vi "Chronos TDMS File Viewer GUI.vi"(9 "ID":string, 10 "Default Time":T1, 11 "Default Channels":string[](array[string])) -> ()   [LabVIEW 2021]
uses:
  Viewer/cluster CC Channel from TDMS.ctl
  typedefs/Chronos cluster GUI Settings.ctl
  <vilib>/Utility/miscctls.llb/LVRangeTypeDef.ctl
  typedefs/Chronos cluster Current File.ctl
  typedefs/Chronos cluster Time Ranges.ctl
  Viewer/Chronos cluster Plot Settings.ctl
  GUI/Chronos cluster Map Limit Plots.ctl
  typedefs/Chronos cluster Plot Data and Limits.ctl
panel:
  in  "Channel Select":i32[](listbox)
  in  "reload":bool
  in  "Log Y":bool
  in  "Legend Visible":enum8{"False", "True", "Mixed"}(c332)
  in  "Y Autoscale":bool
  in  "X Autoscale":bool
  out "Loading...":string="LOADING..."
  out "XY Graph":cluster{dbl[], dbl[]}[](graph)
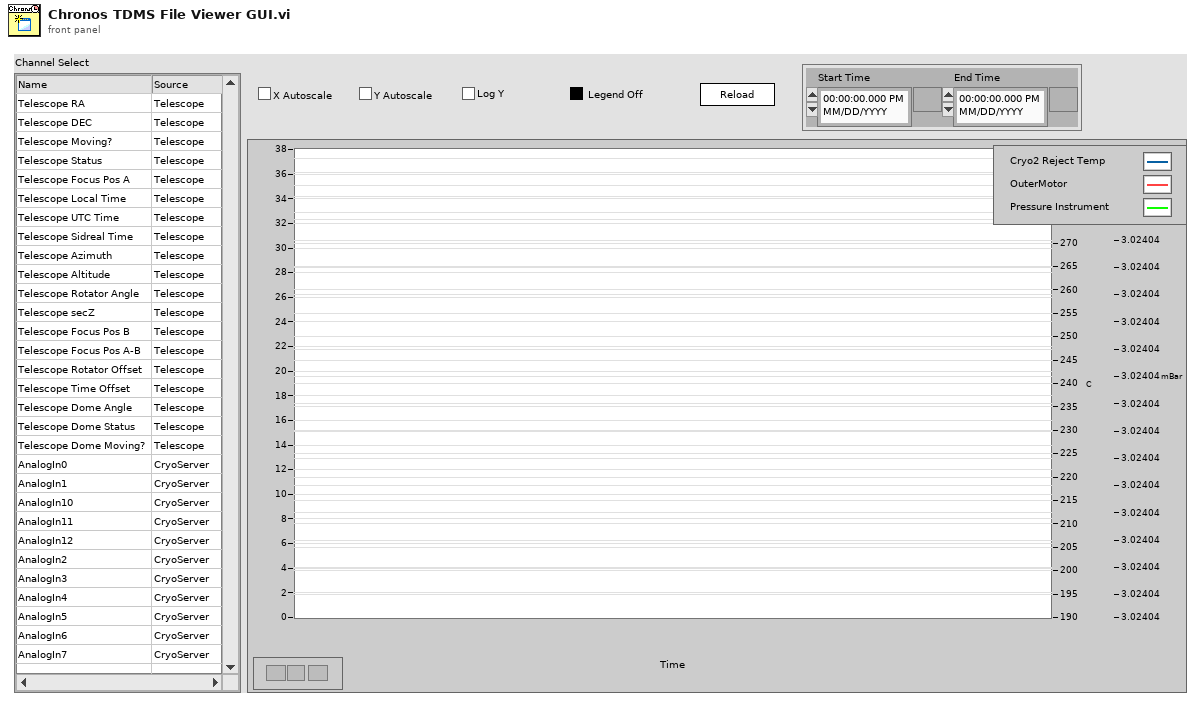
[diagram p1: front panel]
types:
  T1 = cluster{"Start Time":timestamp, "End Time":timestamp}
  T2 = typedef "cluster CC Channel from TDMS.ctl" = cluster{"Name":string, "Source":string, "Units":string}
  T3 = typedef "Chronos cluster GUI Settings.ctl" = cluster{"X Range":T4, "Select Ch":string[], "AutoScale":bool, "Show Limits":bool, "Path":path}
  T4 = typedef "LVRangeTypeDef.ctl" = cluster{"Minimum":dbl, "Maximum":dbl, "Increment":dbl, "Minor Increment":dbl, "Start":dbl}
  T5 = typedef "Chronos cluster Current File.ctl" = cluster{"path":path, "size":i64, "Plot Names":string[], "Offset":i32}
  T6 = typedef "Chronos cluster Time Ranges.ctl" = cluster{"Start Time":timestamp[], "End Time":timestamp[]}
  T7 = typedef "Chronos cluster Plot Settings.ctl" = cluster{"Plot Names":string[], "Colors":u32[], "Y Axis Indecies":i32[], "Units":string[], "Line Style":u8[]}
  T8 = typedef "Chronos cluster Map Limit Plots.ctl" = map{string, T9}
  T9 = typedef "Chronos cluster Plot Data and Limits.ctl" = cluster{"Data":cluster{dbl[], dbl[]}, "Data Units":string, "Limits":cluster{dbl[], dbl[]}[], "Limit Names":string[], "Channel":T2, "Group":string}
  T10 = cluster{"state":refnum<user-event>, "TDMS Files":path[], "Channel Names":string[], "Ch Data":T2[], "Settings":T3, "Current File":T5, "Time Ranges":T6, "Default Channels":string[], "Default Time":cluster{"Start Time":timestamp, "End Time":timestamp}, "Plot Attribs":T7, "Legend":enum8{"False", "True", "Mixed"}, "Plot":T8, "ID":string, "ch":T2}
  T11 = enum16{"open", "open or create", "create or replace", "create", "open (read-only)"}
  T12 = typedef "LVRectTypeDef.ctl" = cluster{"Left":i16, "Top":i16, "Right":i16, "Bottom":i16}
  T13 = typedef "Chronos cluster Viewer Window.ctl" = cluster{"Bounds":T12, "Channels":string[]}
  T14 = typedef "Chronos map Viewer Window List.ctl" = map{string, T13}
  T15 = enum32{"invalid app kind", "Development System", "Run Time System", "Student Edition", "Embedded LabVIEW", "Evaluation", "Custom"}
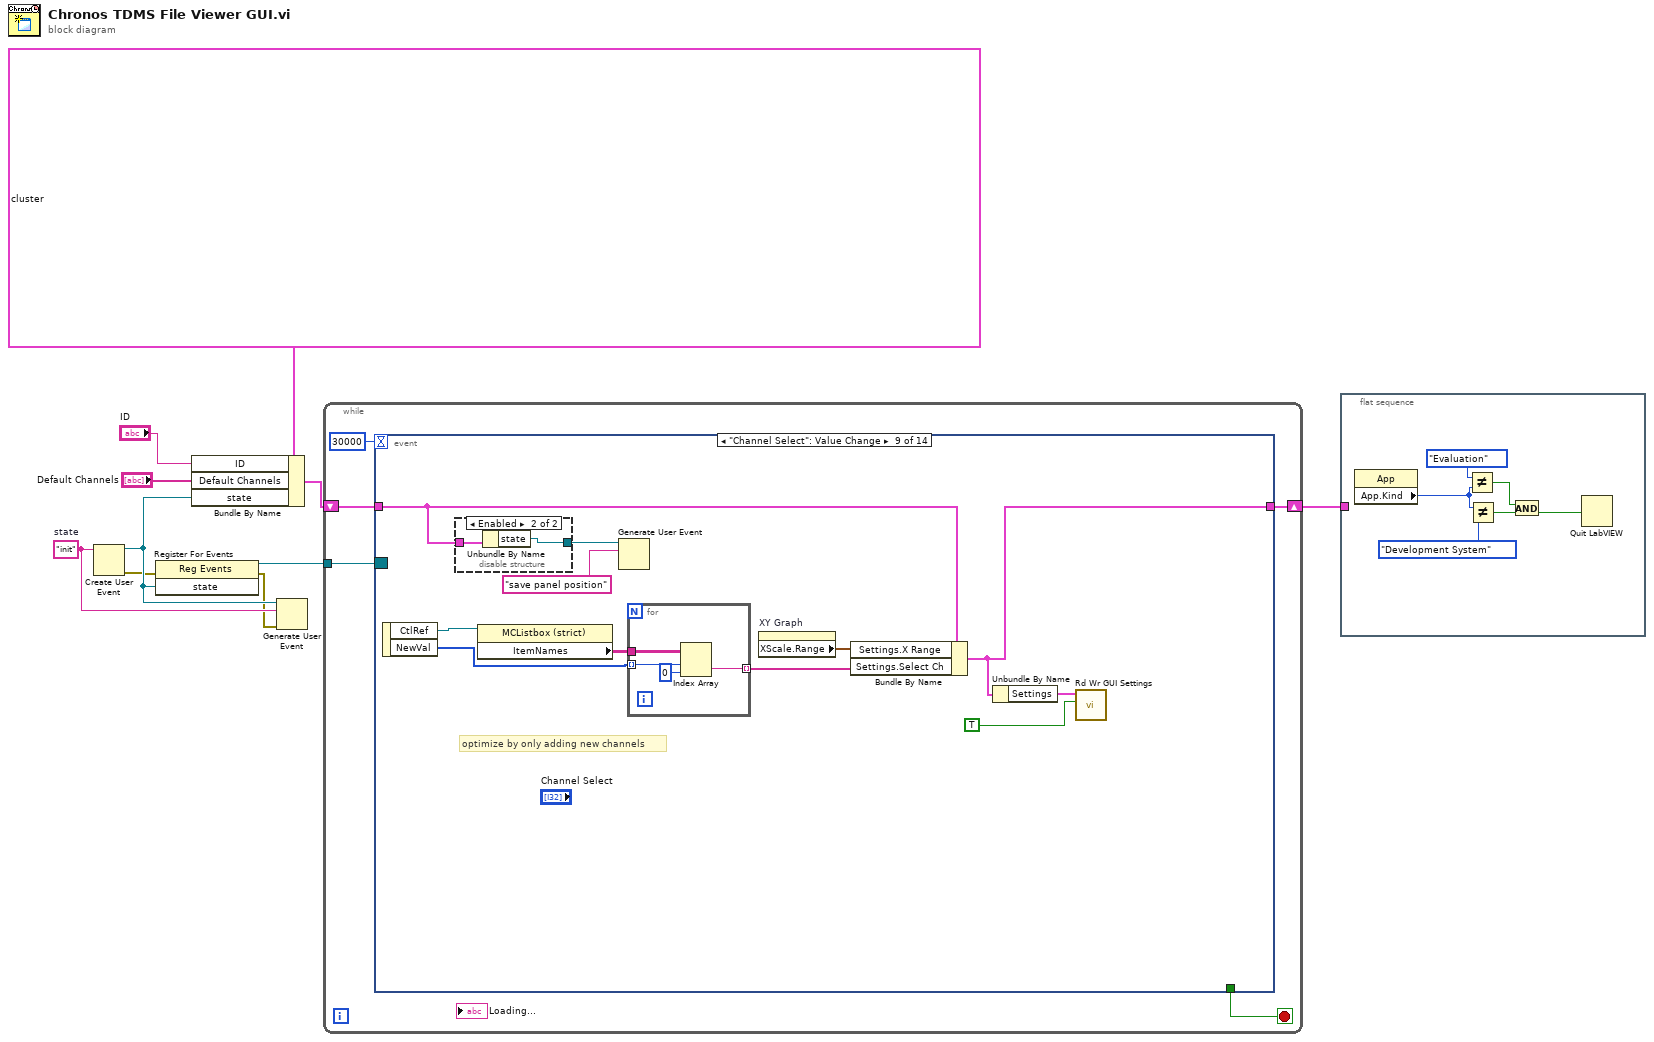
[diagram p0: block diagram]
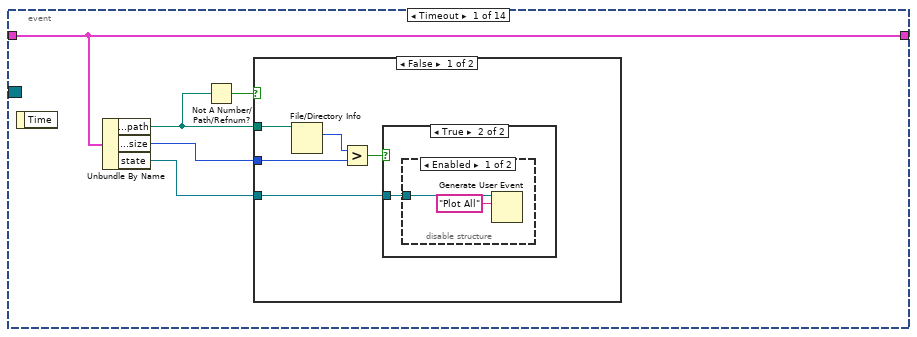
[diagram p2: hidden frame]
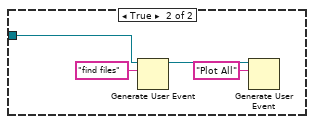
[diagram p5: hidden frame]
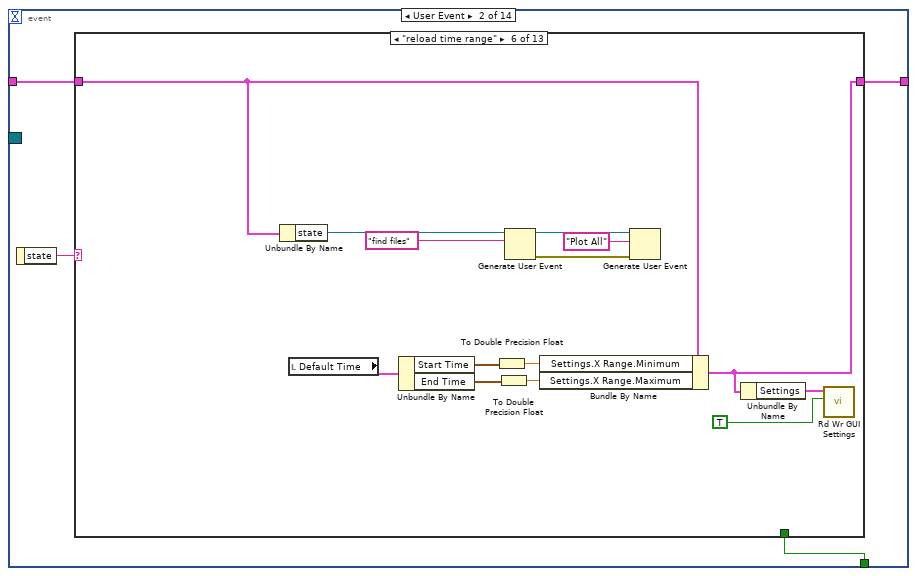
[diagram p6: hidden frame]
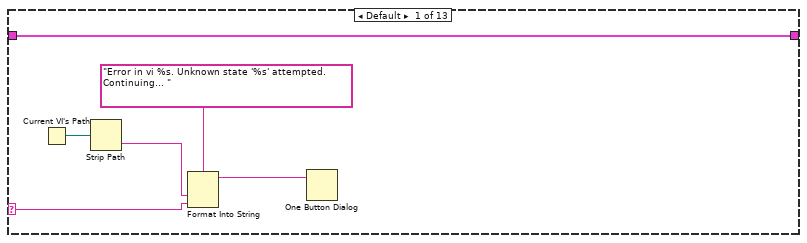
[diagram p7: hidden frame]
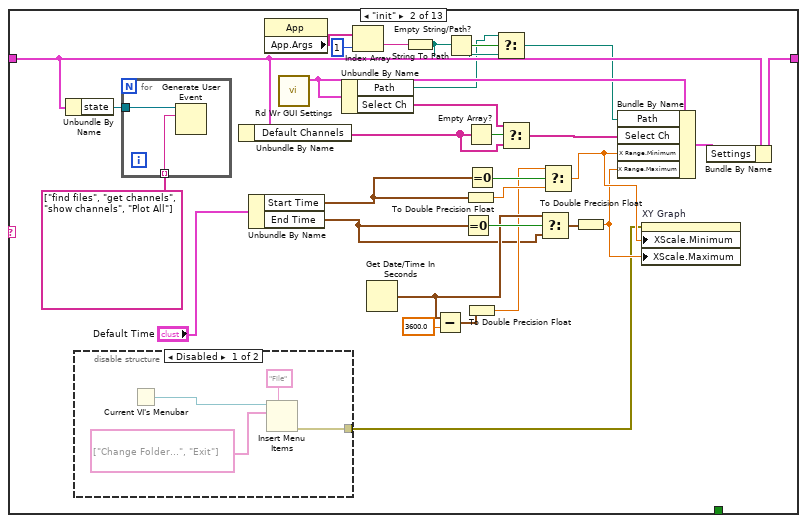
[diagram p8: hidden frame]
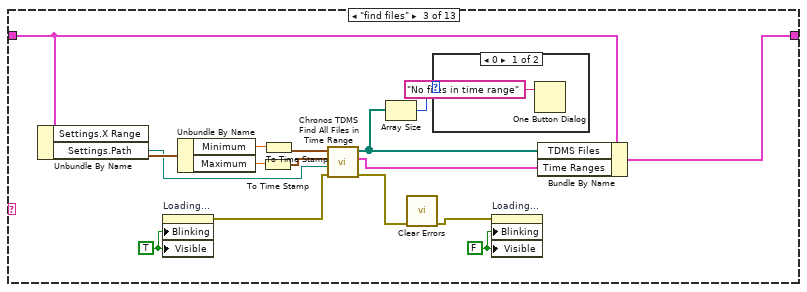
[diagram p10: hidden frame]
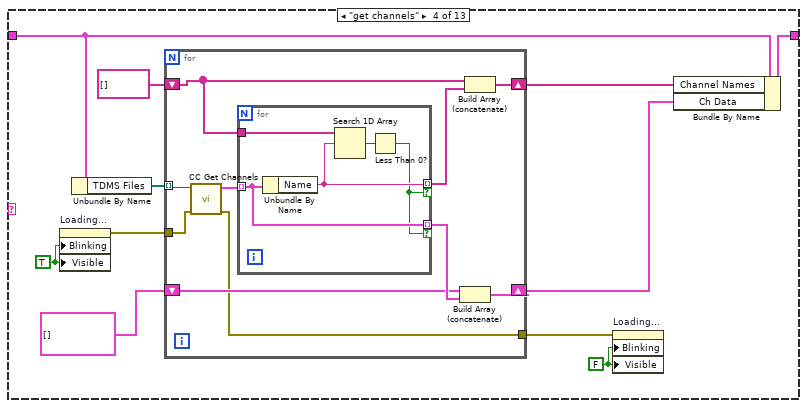
[diagram p12: hidden frame]
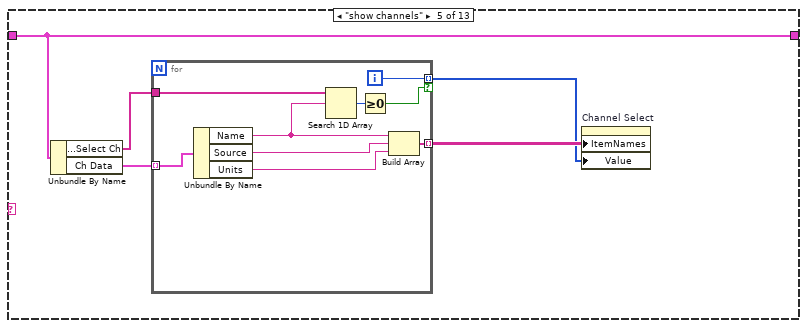
[diagram p13: hidden frame]
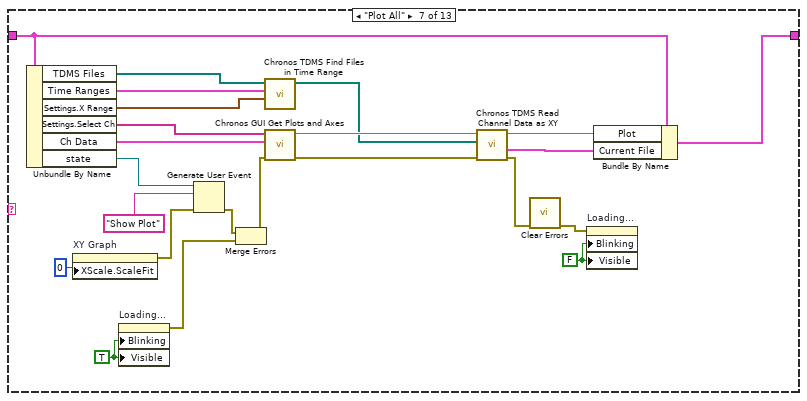
[diagram p14: hidden frame]
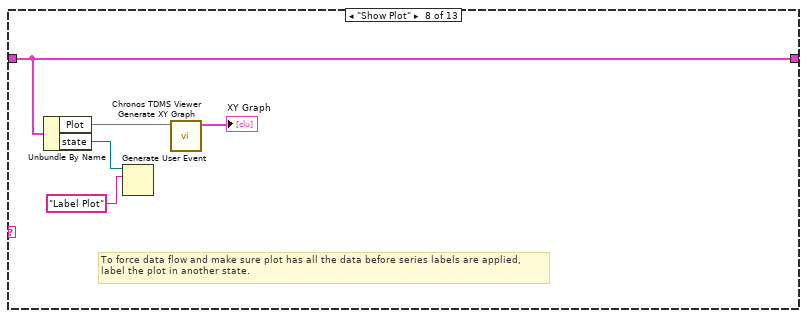
[diagram p15: hidden frame]
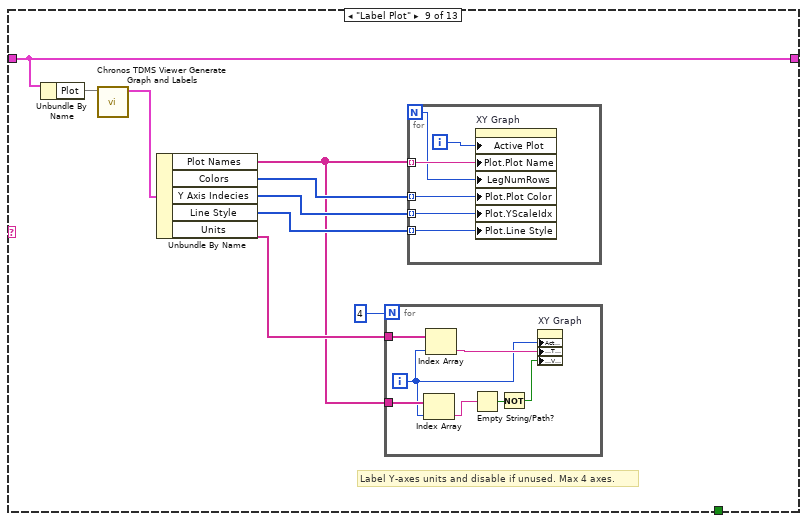
[diagram p16: hidden frame]
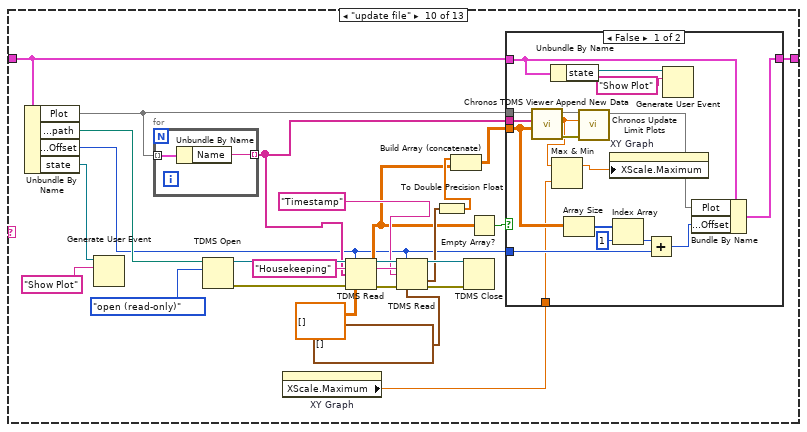
[diagram p17: hidden frame]
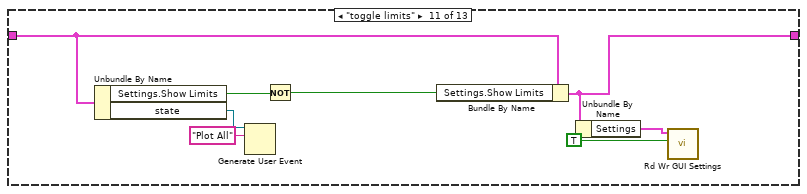
[diagram p19: hidden frame]
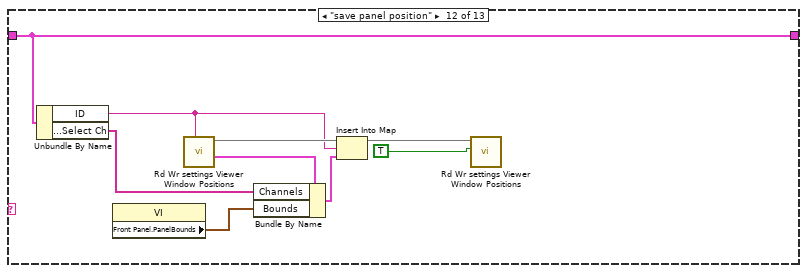
[diagram p20: hidden frame]
diagram:
  w6 = "init"  # state
  n1 = Create User Event(user event datatype=w6) -> (user event=w8:refnum<user-event>, error out=w4:errorcluster)  [unwired: 1 in]
  n2 = register-events(error in=w4, w8) -> (reference out=w7:refnum<event-registration>, error out=w5:errorcluster)  [unwired: 1 in]
  n3 = Bundle By Name(cluster=T10 {"state"=refnum, "TDMS Files"=[], "Channel Names"=[], "Ch Data"=[], "Settings"={"X Range"={"Minimum"=0.0, "Maximum"=0.0, "Increment"=0.0, "Minor Increment"=0.0, "Start"=0.0}, "Select Ch"=[], "AutoScale"=FALSE, "Show Limits"=FALSE, "Path"=path ""}, "Current File"={"path"=path "", "size"=0, "Plot Names"=[], "Offset"=0}, "Time Ranges"={"Start Time"=[], "End Time"=[]}, "Default Channels"=[], "Default Time"={"Start Time"=timestamp(0 s since 1904-01-01), "End Time"=timestamp(0 s since 1904-01-01)}, "Plot Attribs"={"Plot Names"=["Channel 02", "Channel 02 Red Low", "Channel 02 Red Hi", "Channel 02 Yellow Low", "Channel 02 Yellow Hi", "Channel 1", "Channel 1 Red Low", "Channel 1 Red Hi", "Channel 1 Yellow Low", "Channel 1 Yellow Hi"], "Colors"=[483491, 483491, 483491, 483491, 483491, 16728642, 16728642, 16728642, 16728642, 16728642], "Y Axis Indecies"=[0, 0, 0, 0, 0, 0, 0, 0, 0, 0], "Units"=["V"], "Line Style"=[]}, "Legend"=enum."False", "Plot"={}, "ID"="", "ch"={"Name"="", "Source"="", "Units"=""}}, "ID"="ID", "Default Channels"="Default Channels", "state"=w8) -> (w9:T10)
  n4 = Generate User Event(user event=w8, event data cluster=w6, error in=w5) -> ()  [unwired: 1 in, 2 out]
  n5 = while {
    tunnel: w7 -> [w15]
    shift-right: [w13] -> w1
    shift-left: w9 -> [w14]
    stop <- w12 stop-if-true
    n6 = event shown="[8] \"Channel Select\": Value Change" {
      selector: w15 -> [_ _ _ _ _ _ _ _ _ _ _ _ _ _]
      dyn-events: _ -> [_ _ _ _ _ _ _ _ _ _ _ _ _ _]
      timeout: 30000 -> [_ _ _ _ _ _ _ _ _ _ _ _ _ _]
      tunnel: w14 -> [w20 w35 w274 w313 w316 w318 w323 w327 w354 w374 w379 w385 w387 w393]
      tunnel: [w20 w34 w275 w313 w316 w318 w323 w328 w351 w374 w379 w385 w388 w393] -> w13
      tunnel: [_ w33 _ _ _ _ _ _ _ _ _ _ _ TRUE ("Close")] -> w12
      event Timeout {
        n7 = event-data() -> ()  [unwired: 1 in, 1 out]
        n8 = Unbundle By Name(w20) -> ("Current File.path"=w18:path, "Current File.size"=w17:i64, "state"=w16:refnum<user-event>)
        n9 = Not A Number/Path/Refnum?(number/path/refnum=w18) -> (NaN/Path/Refnum?=w19:bool)
        n10 = case shown="False" w19 {
          tunnel: w18 -> [w25 _]
          tunnel: w17 -> [w23 _]
          tunnel: w16 -> [w22 w31]
          frame False {
            n11 = File/Directory Info(path=w25) -> (size=w24:i64)  [unwired: 1 in, 6 out]
            n12 = Greater?(x=w24, y=w23) -> (0:w21:bool)
            n13 = case shown="True" w21 {
              tunnel: w22 -> [_ w26]
              frame False {
              }
              frame True {
                n14 = disable-structure shown="Enabled" {
                  disable-tunnel: w26 -> [w28 _]
                  frame Enabled {
                    n15 = Generate User Event(user event=w28, event data cluster="Plot All" ("event data")) -> ()  [unwired: 2 in, 2 out]
                  }
                  frame Disabled {
                  }
                }
              }
            }
          }
          frame True {
            n16 = Generate User Event(user event=w31, event data cluster="find files" ("event data")) -> (user event out=w30:refnum<user-event>)  [unwired: 2 in, 1 out]
            n17 = Generate User Event(user event=w30, event data cluster="Plot All" ("event data")) -> ()  [unwired: 2 in, 2 out]
          }
        }
      }
      event User Event {
        n18 = event-data() -> ("state"=w36:string)  [unwired: 1 in]
        n19 = case shown="\"reload time range\"" w36 {
          selector: w36 -> [w41 _ _ _ _ _ _ _ _ _ _ _ _]
          tunnel: w35 -> [w37 w69 w94 w104 w127 w143 w171 w178 w181 w218 w248 w263 w265]
          tunnel: [w37 w71 w95 w105 w127 w142 w172 w178 w181 w219 w249 w263 w265] -> w34
          tunnel: [_ _ _ _ _ _ _ _ _ _ _ _ TRUE] -> w33
          frame Default {
            n20 = Current VI's Path() -> (path=w40:path)
            n21 = Strip Path(path=w40) -> (name=w39:string)  [unwired: 1 out]
            n22 = Format Into String(format string="Error in vi %s. Unknown state '%s' attempted. Continuing... ", w39, w41) -> (resulting string=w38:string)  [unwired: 2 in, 1 out]
            n23 = One Button Dialog(message=w38) -> ()  [unwired: 1 in, 1 out]
          }
          frame "init" {
            n24 = Unbundle By Name(w69) -> ("state"=w73:refnum<user-event>)
            n25 = disable-structure shown="Disabled" {
              disable-tunnel: [w74 _] -> w43
              frame Disabled {
                n26 = Current VI's Menubar() -> (w77:refnum<k9>)
                n27 = Insert Menu Items(5:"File" ("menu tag"), 8:string[] ["Change Folder...", "Exit"] ("item names"), 9:w77) -> (0:w74:errorcluster)  [unwired: 3 in, 2 out]
              }
              frame Enabled {
              }
            }
            n28 = for {
              tunnel: w73 -> [w79]
              tunnel: string[] ["find files", "get channels", "show channels", "Plot All"] -> [w78] mode=indexing
              n29 = Generate User Event(user event=w79, event data cluster=w78) -> ()  [unwired: 2 in, 2 out]
            }
            n30 = Unbundle By Name(w69) -> ("Default Channels"=w64:string[])
            n31 = Unbundle By Name("Default Time") -> ("Start Time"=w45:timestamp, "End Time"=w44:timestamp)
            n32 = property class="App"() -> ("App.Args"=w53:string[])  [unwired: 2 in, 2 out]
            n33 = call "Rd Wr GUI Settings.vi"() -> ("Settings"=w68:T3)  [unwired: 10 in, 1 out]
            n34 = Unbundle By Name(w68) -> ("Path"=w49:path, "Select Ch"=w66:string[])
            n35 = Index Array(array=w53, index=1) -> (element=w51:string)
            n36 = Get Date/Time In Seconds() -> (seconds since 1Jan1904=w57:timestamp)
            n37 = String To Path(string=w51) -> (path=w50:path)
            n38 = Subtract(x=w57, y=3600.0) -> (x-y=w55:timestamp)
            n39 = Empty String/Path?(string/path=w50) -> (empty?=w52:bool)
            n40 = Equal To 0?(x=w44) -> (x = 0?=w62:bool)
            n41 = Empty Array?(array=w64) -> (empty?=w67:bool)
            n42 = To Double Precision Float(number=w45) -> (double precision float=w60:dbl)
            n43 = Equal To 0?(x=w45) -> (x = 0?=w63:bool)
            n44 = To Double Precision Float(number=w55) -> (double precision float=w54:dbl)
            n45 = Select(t=w49, s=w52, f=w50) -> (s? t:f=w48:path)
            n46 = Select(t=w66, s=w67, f=w64) -> (s? t:f=w65:string[])
            n47 = Select(t=w57, s=w62, f=w44) -> (s? t:f=w61:timestamp)
            n48 = Select(t=w54, s=w63, f=w60) -> (s? t:f=w59:dbl)
            n49 = To Double Precision Float(number=w61) -> (double precision float=w58:dbl)
            n50 = Bundle By Name(cluster=w68, "Path"=w48, "Select Ch"=w65, "X Range.Minimum"=w59, "X Range.Maximum"=w58) -> (w70:T3)
            n51 = property on="XY Graph" class="XYGraph (strict)"(error in=w43, "XScale.Minimum"=w59, "XScale.Maximum"=w58) -> ()  [unwired: 1 in, 2 out]
            n52 = Bundle By Name(cluster=w69, "Settings"=w70) -> (w71:T10)
          }
          frame "find files" {
            w85 = FALSE ("Visible")
            w87 = TRUE ("Visible")
            n53 = Unbundle By Name(w94) -> ("Settings.X Range"=w89:T4, "Settings.Path"=w82:path)
            n54 = property on="Loading..." class="Str"("Blinking"=w87, "Visible"=w87) -> (error out=w86:errorcluster)  [unwired: 2 in, 1 out]
            n55 = Unbundle By Name(w89) -> ("Minimum"=w93:dbl, "Maximum"=w92:dbl)
            n56 = To Time Stamp(1:w92) -> (0:w90:timestamp)
            n57 = To Time Stamp(1:w93) -> (0:w91:timestamp)
            n58 = call "Chronos TDMS Find All Files in Time Range.vi"("error in (no error)"=w86, "path"=w82, "End Time"=w90, "Start Time"=w91) -> ("error out"=w84:errorcluster, "Time Ranges"=w88:T6, "Files"=w81:path[])  [unwired: 5 in]
            n59 = Array Size(array=w81) -> (size(s)=w80:i32)
            n60 = call <vilib>:"Clear Errors.vi"("error in (no error)"=w84) -> ("error out"=w83:errorcluster)  [unwired: 5 in, 1 out]
            n61 = case shown="0" w80 {
              frame 0 {
                n62 = One Button Dialog(message="No files in time range") -> ()  [unwired: 1 in, 1 out]
              }
              frame 1, Default {
              }
            }
            n63 = property on="Loading..." class="Str"(error in=w83, "Blinking"=w85, "Visible"=w85) -> ()  [unwired: 1 in, 2 out]
            n64 = Bundle By Name(cluster=w94, "TDMS Files"=w81, "Time Ranges"=w88) -> (w95:T10)
          }
          frame "get channels" {
            w98 = FALSE ("Visible")
            w100 = TRUE ("Visible")
            n65 = property on="Loading..." class="Str"("Blinking"=w100, "Visible"=w100) -> (error out=w99:errorcluster)  [unwired: 2 in, 1 out]
            n66 = Unbundle By Name(w104) -> ("TDMS Files"=w107:path[])
            n67 = for {
              tunnel: w107 -> [w111] mode=indexing
              shift-right: [w117] -> w103
              shift-left: string[] [] -> [w116]
              shift-right: [w114] -> w101
              shift-left: T2[] [] -> [w112]
              tunnel: w99 -> [w109]
              tunnel: [w108] -> w97
              n68 = call "CC Get Channels.vi"("error in (no error)"=w109, "file path"=w111) -> ("error out"=w108:errorcluster, "Channel List"=w110:T2[])  [unwired: 8 in]
              n69 = for {
                tunnel: w110 -> [w119] mode=indexing
                tunnel: w116 -> [w122]
                tunnel: [w120] -> w115 mode=indexing if=w118
                tunnel: [w119] -> w113 mode=indexing if=w118
                n70 = Unbundle By Name(w119) -> ("Name"=w120:string)
                n71 = Search 1D Array(1D array=w122, element=w120) -> (index of element=w121:i32)  [unwired: 1 in]
                n72 = Less Than 0?(x=w121) -> (x < 0?=w118:bool)
              }
              n73 = Build Array (concatenate)(w112, w113) -> (w114:T2[])
              n74 = Build Array (concatenate)(w116, w115) -> (w117:string[])
            }
            n75 = property on="Loading..." class="Str"(error in=w97, "Blinking"=w98, "Visible"=w98) -> ()  [unwired: 1 in, 2 out]
            n76 = Bundle By Name(cluster=w104, "Channel Names"=w103, "Ch Data"=w101) -> (w105:T10)
          }
          frame "show channels" {
            n77 = Unbundle By Name(w127) -> ("Settings.Select Ch"=w124:string[], "Ch Data"=w126:T2[])
            n78 = for {
              tunnel: w126 -> [w136] mode=indexing
              tunnel: [w135] -> w125 mode=indexing
              tunnel: w124 -> [w134]
              tunnel: [w131] -> w123 mode=indexing if=w130
              i -> [w131]
              n79 = Unbundle By Name(w136) -> ("Name"=w133:string, "Source"=w129:string, "Units"=w128:string)
              n80 = Search 1D Array(1D array=w134, element=w133) -> (index of element=w132:i32)  [unwired: 1 in]
              n81 = Greater Or Equal To 0?(x=w132) -> (x >= 0?=w130:bool)
              n82 = Build Array(w133, w129, w128) -> (w135:string[])
            }
            n83 = property on="Channel Select" class="MCListbox (strict)"("ItemNames"=w125, "Value"=w123) -> ()  [unwired: 2 in, 2 out]
          }
          frame "reload time range" {
            n84 = Unbundle By Name(w143) -> ("state"=w148:refnum<user-event>)
            n85 = local read "Default Time"() -> (w141:T1)
            n86 = Unbundle By Name(w141) -> ("Start Time"=w139:timestamp, "End Time"=w138:timestamp)
            n87 = To Double Precision Float(number=w139) -> (double precision float=w140:dbl)
            n88 = To Double Precision Float(number=w138) -> (double precision float=w137:dbl)
            n89 = Generate User Event(user event=w148, event data cluster="find files" ("event data")) -> (user event out=w146:refnum<user-event>, error out=w145:errorcluster)  [unwired: 2 in]
            n90 = Bundle By Name(cluster=w143, "Settings.X Range.Minimum"=w140, "Settings.X Range.Maximum"=w137) -> (w142:T10)
            n91 = Generate User Event(user event=w146, event data cluster="Plot All" ("event data"), error in=w145) -> ()  [unwired: 1 in, 2 out]
            n92 = Unbundle By Name(w142) -> ("Settings"=w150:T3)
            n93 = call "Rd Wr GUI Settings.vi"("Write? (F:Read)"=TRUE, "Settings"=w150) -> ()  [unwired: 8 in, 2 out]
          }
          frame "Plot All" {
            w153 = FALSE ("Visible")
            w157 = TRUE ("Visible")
            n94 = Unbundle By Name(w171) -> ("TDMS Files"=w173:path[], "Time Ranges"=w170:T6, "Settings.X Range"=w167:T4, "Settings.Select Ch"=w169:string[], "Ch Data"=w168:T2[], "state"=w166:refnum<user-event>)
            n95 = property on="XY Graph" class="XYGraph (strict)"("XScale.ScaleFit"=u8 0 ("X Scale.Scale Fit")) -> (error out=w159:errorcluster)  [unwired: 2 in, 1 out]
            n96 = property on="Loading..." class="Str"("Blinking"=w157, "Visible"=w157) -> (error out=w154:errorcluster)  [unwired: 2 in, 1 out]
            n97 = Generate User Event(user event=w166, event data cluster="Show Plot" ("event data"), error in=w159) -> (error out=w156:errorcluster)  [unwired: 1 in, 1 out]
            n98 = Merge Errors(w156, w154) -> (w155:errorcluster)
            n99 = call "Chronos TDMS Find Files in Time Range.vi"("Scale"=w167, "Time Ranges"=w170, "TDMS Files"=w173) -> ("Files out"=w162:path[])  [unwired: 7 in, 1 out]
            n100 = call "Chronos GUI Get Plots and Axes.vi"("error in (no error)"=w155, "Ch Data"=w168, "Select Ch"=w169) -> ("error out"=w163:errorcluster, "Plot Map"=w164:T8)  [unwired: 7 in]
            n101 = call "Chronos TDMS Read Channel Data as XY.vi"("error in (no error)"=w163, "Files"=w162, "Limit Plot Map"=w164) -> ("error out"=w152:errorcluster, "Current File"=w160:T5, "Plot Map out"=w161:T8)  [unwired: 6 in]
            n102 = call <vilib>:"Clear Errors.vi"("error in (no error)"=w152) -> ("error out"=w151:errorcluster)  [unwired: 5 in, 1 out]
            n103 = property on="Loading..." class="Str"(error in=w151, "Blinking"=w153, "Visible"=w153) -> ()  [unwired: 1 in, 2 out]
            n104 = Bundle By Name(cluster=w171, "Plot"=w161, "Current File"=w160) -> (w172:T10)
          }
          frame "Show Plot" {
            # "To force data flow and make sure plot has all the data before series labels are applied,\nlabel the plot in another state."
            n105 = Unbundle By Name(w178) -> ("Plot"=w175:T8, "state"=w177:refnum<user-event>)
            n106 = Generate User Event(user event=w177, event data cluster="Label Plot" ("event data")) -> ()  [unwired: 2 in, 2 out]
            n107 = call "Chronos TDMS Viewer Generate XY Graph.vi"("Limit Plot Map"=w175) -> ("XY Graph"=→"XY Graph":cluster{dbl[], dbl[]}[])  [unwired: 9 in, 1 out]
          }
          frame "Label Plot" {
            # "Label Y-axes units and disable if unused. Max 4 axes."
            n108 = Unbundle By Name(w181) -> ("Plot"=w182:T8)
            n109 = call "Chronos TDMS Viewer Generate Graph and Labels.vi"("Limit Plot Map"=w182) -> ("Plot Settings"=w180:T7)  [unwired: 9 in, 1 out]
            n110 = Unbundle By Name(w180) -> ("Plot Names"=w179:string[], "Colors"=w187:u32[], "Y Axis Indecies"=w186:i32[], "Line Style"=w184:u8[], "Units"=w185:string[])
            n111 = for {
              N: 4 -> [_]
              tunnel: w185 -> [w193]
              tunnel: w179 -> [w190]
              i -> [w189]
              n112 = Index Array(array=w190, index=w189) -> (element=w188:string)
              n113 = Index Array(array=w193, index=w189) -> (element=w194:string)
              n114 = Empty String/Path?(string/path=w188) -> (empty?=w192:bool)
              n115 = Not(x=w192) -> (.not. x?=w191:bool)
              n116 = property on="XY Graph" class="XYGraph (strict)"("ActYScl"=w189, "YScale.NameLbl.Text"=w194, "YScale.Visible"=w191) -> ()  [unwired: 2 in, 2 out]
            }
            n117 = for {
              N -> [w198]
              tunnel: w179 -> [w199] mode=indexing
              tunnel: w186 -> [w197] mode=indexing
              tunnel: w187 -> [w196] mode=indexing
              tunnel: w184 -> [w195] mode=indexing
              i -> [w200]
              n118 = property on="XY Graph" class="XYGraph (strict)"("Active Plot"=w200, "Plot.Plot Name"=w199, "LegNumRows"=w198, "Plot.Plot Color"=w196, "Plot.YScaleIdx"=w197, "Plot.Line Style"=w195) -> ()  [unwired: 2 in, 2 out]
            }
          }
          frame "update file" {
            n119 = Unbundle By Name(w218) -> ("Plot"=w220:T8, "Current File.path"=w225:path, "Current File.Offset"=w201:i32, "state"=w217:refnum<user-event>)
            n120 = Generate User Event(user event=w217, event data cluster="Show Plot" ("event data")) -> ()  [unwired: 2 in, 2 out]
            n121 = for {
              tunnel: w220 -> [w247] mode=indexing
              tunnel: [w246] -> w213 mode=indexing
              n122 = Unbundle By Name(w247) -> ("Name"=w246:string)
            }
            n123 = TDMS Open(10:T11."open (read-only)" ("operation (0:open)"), 11:w225) -> (0:w222:errorcluster, 3:w223:refnum<k34>)  [unwired: 5 in]
            n124 = property on="XY Graph" class="XYGraph (strict)"() -> ("XScale.Maximum"=w214:dbl)  [unwired: 2 in, 2 out]
            n125 = TDMS Read(0:w223, 1:w201, 5:"Housekeeping" ("group name in"), 7:w213, 11:w222, 12:dbl[][] []) -> (4:w212:refnum<k34>, 6:w211:string, 10:w203:dbl[][], 15:w210:errorcluster)  [unwired: 2 in, 2 out]
            n126 = TDMS Read(0:w212, 1:w201, 5:w211, 7:"Timestamp", 11:w210, 12:timestamp[] []) -> (4:w206:refnum<k34>, 10:w205:timestamp[], 15:w207:errorcluster)  [unwired: 2 in, 3 out]
            n127 = To Double Precision Float(number=w205) -> (double precision float=w204:dbl[])
            n128 = Build Array (concatenate)(w204, w203) -> (w202:dbl[][])
            n129 = TDMS Close(8:w207, 11:w206) -> ()  [unwired: 2 out]
            n130 = Empty Array?(array=w203) -> (empty?=w215:bool)
            n131 = case shown="False" w215 {
              tunnel: w220 -> [w244 _]
              tunnel: [w241 w245] -> w219
              tunnel: w218 -> [w234 w245]
              tunnel: w201 -> [w239 _]
              tunnel: w202 -> [w236 _]
              tunnel: w213 -> [w231 _]
              tunnel: w214 -> [w228 _]
              frame False {
                n132 = call "Chronos TDMS Viewer Append New Data.vi"("data"=w236, "Ch Names"=w231, "Plot"=w244) -> ("error out"=w243:errorcluster, "end time"=w230:dbl, "Plot out"=w242:T8)  [unwired: 6 in]
                n133 = Unbundle By Name(w234) -> ("state"=w233:refnum<user-event>)
                n134 = Max & Min(x=w230, y=w228) -> (max(x,y)=w229:dbl)  [unwired: 1 out]
                n135 = Array Size(array=w236) -> (size(s)=w240:i32[])
                n136 = call "Chronos Update Limit Plots.vi"("error in (no error)"=w243, "End Time"=w230, "Limits"=w242) -> ("Limits out"=w235:T8)  [unwired: 7 in, 1 out]
                n137 = property on="XY Graph" class="XYGraph (strict)"("XScale.Maximum"=w229) -> ()  [unwired: 2 in, 2 out]
                n138 = Index Array(array=w240, index=1) -> (element=w227:i32)
                n139 = Add(x=w227, y=w239) -> (x+y=w238:i32)
                n140 = Generate User Event(user event=w233, event data cluster="Show Plot" ("event data")) -> ()  [unwired: 2 in, 2 out]
                n141 = Bundle By Name(cluster=w234, "Plot"=w235, "Current File.Offset"=w238) -> (w241:T10)
              }
              frame True {
              }
            }
          }
          frame "toggle limits" {
            n142 = Unbundle By Name(w248) -> ("Settings.Show Limits"=w255:bool, "state"=w253:refnum<user-event>)
            n143 = Generate User Event(user event=w253, event data cluster="Plot All" ("event data")) -> ()  [unwired: 2 in, 2 out]
            n144 = Not(x=w255) -> (.not. x?=w254:bool)
            n145 = Bundle By Name(cluster=w248, "Settings.Show Limits"=w254) -> (w249:T10)
            n146 = Unbundle By Name(w249) -> ("Settings"=w251:T3)
            n147 = call "Rd Wr GUI Settings.vi"("Write? (F:Read)"=TRUE, "Settings"=w251) -> ()  [unwired: 8 in, 2 out]
          }
          frame "save panel position" {
            n148 = Unbundle By Name(w263) -> ("ID"=w262:string, "Settings.Select Ch"=w259:string[])
            n149 = property class="VI"() -> ("Front Panel.PanelBounds"=w260:T12)  [unwired: 2 in, 2 out]
            n150 = call "Rd Wr settings Viewer Window Positions.vi"("Window name"=w262) -> ("value"=w261:T13, "Window Map"=w264:T14)  [unwired: 7 in, 2 out]
            n151 = Bundle By Name(cluster=w261, "Channels"=w259, "Bounds"=w260) -> (w256:T13)
            n152 = Insert Into Map(map in=w264, key=w262, value=w256) -> (map out=w258:T14)  [unwired: 2 out]
            n153 = call "Rd Wr settings Viewer Window Positions.vi"("Write? (F:Read)"=TRUE, "Window Map"=w258) -> ()  [unwired: 6 in, 4 out]
          }
          frame "shutdown" {
            n154 = Unbundle By Name(w265) -> ("ID"=w267:string)
            n155 = call "Rd Wr settings Viewer Window Positions.vi"("Window name"=w267) -> ("Not Found?"=w266:bool, "Window Map"=w268:T14)  [unwired: 7 in, 2 out]
            n156 = case shown="False" w266 {
              tunnel: w268 -> [w271 _]
              tunnel: w267 -> [w270 _]
              frame False {
                n157 = Remove From Map(10:w270, 11:w271) -> (3:w273:T14)  [unwired: 2 out]
                n158 = call "Rd Wr settings Viewer Window Positions.vi"("Write? (F:Read)"=TRUE, "Window Map"=w273) -> ()  [unwired: 6 in, 4 out]
              }
              frame True {
              }
            }
          }
        }
      }
      event Menu Selection (User) {
        n159 = event-data() -> ("MenuRef"=w276:refnum<k9>, "ItemTag"=w277:string)  [unwired: 1 in, 5 out]
        n160 = case shown="\"False\", Default" w277 {
          selector: w277 -> [_ w285 _ _]
          tunnel: w274 -> [_ w289 w292 w309]
          tunnel: w276 -> [_ w286 _ _]
          tunnel: w274 -> [w278 w287 w295 w310]
          tunnel: [w278 w282 w293 w310] -> w275
          frame "False", Default {
          }
          frame "Show Limits" {
            n161 = Unbundle By Name(w289) -> ("Settings.Show Limits"=w288:bool, "state"=w284:refnum<user-event>)
            n162 = Generate User Event(user event=w284, event data cluster="Plot All" ("event data")) -> ()  [unwired: 2 in, 2 out]
            n163 = Not(x=w288) -> (.not. x?=w279:bool)
            n164 = Set Menu Item Info(6:w279, 7:w285, 11:w286) -> ()  [unwired: 4 in, 2 out]
            n165 = Bundle By Name(cluster=w287, "Settings.Show Limits"=w279) -> (w282:T10)
            n166 = Unbundle By Name(w282) -> ("Settings"=w281:T3)
            n167 = call "Rd Wr GUI Settings.vi"("Write? (F:Read)"=TRUE, "Settings"=w281) -> ()  [unwired: 8 in, 2 out]
          }
          frame "Change Folder..." {
            n168 = Unbundle By Name(w292) -> ("state"=w291:refnum<user-event>)
            n169 = call "File Dialog"() -> ("selected path"=w294:path, "cancelled"=w296:bool)  [unwired: 12 in, 2 out]
            n170 = case shown="False" w296 {
              tunnel: w295 -> [w303 w306]
              tunnel: w294 -> [w302 _]
              tunnel: [w300 w306] -> w293
              tunnel: w291 -> [w301 _]
              tunnel: string[] ["find files", "get channels", "show channels", "Plot All"] -> [w297 _]
              frame False {
                n171 = for {
                  tunnel: w301 -> [w305]
                  tunnel: w297 -> [w304] mode=indexing
                  n172 = Generate User Event(user event=w305, event data cluster=w304) -> ()  [unwired: 2 in, 2 out]
                }
                n173 = Bundle By Name(cluster=w303, "Settings.Path"=w302) -> (w300:T10)
                n174 = Unbundle By Name(w300) -> ("Settings"=w299:T3)
                n175 = call "Rd Wr GUI Settings.vi"("Write? (F:Read)"=TRUE, "Settings"=w299) -> ()  [unwired: 8 in, 2 out]
              }
              frame True {
              }
            }
          }
          frame "Exit" {
            n176 = Unbundle By Name(w309) -> ("state"=w308:refnum<user-event>)
            n177 = Generate User Event(user event=w308, event data cluster="shutdown" ("event data")) -> ()  [unwired: 2 in, 2 out]
          }
        }
      }
      event Panel Resize {
        n178 = event-data() -> ()  [unwired: 1 in, 6 out]
        n179 = Unbundle By Name(w313) -> ("state"=w312:refnum<user-event>)
        n180 = Generate User Event(user event=w312, event data cluster="save panel position" ("event data")) -> ()  [unwired: 2 in, 2 out]
      }
      event "reload": Value Change {
        n181 = event-data() -> ()  [unwired: 1 in, 6 out]
        n182 = Unbundle By Name(w316) -> ("state"=w315:refnum<user-event>)
        n183 = Generate User Event(user event=w315, event data cluster="reload time range" ("event data")) -> ()  [unwired: 2 in, 2 out]
      }
      event "XY Graph": Mouse Enter {
        n184 = event-data() -> ("CtlRef"=w319:refnum<vi>)  [unwired: 1 in, 3 out]
        n185 = Unbundle By Name(w318) -> ("Legend"=w317:enum8{"False", "True", "Mixed"})
        n186 = case shown="\"Mixed\"" w317 {
          tunnel: w319 -> [_ _ w321]
          frame "False", Default {
          }
          frame "True" {
          }
          frame "Mixed" {
            n187 = property class="XYGraph (strict)"(reference=w321, "Legend Visible"=TRUE ("Legend:Visible")) -> ()  [unwired: 1 in, 2 out]
          }
        }
      }
      event "XY Graph": Mouse Leave {
        n188 = event-data() -> ("CtlRef"=w324:refnum<vi>)  [unwired: 1 in, 3 out]
        n189 = Unbundle By Name(w323) -> ("Legend"=w322:enum8{"False", "True", "Mixed"})
        n190 = case shown="\"Mixed\"" w322 {
          tunnel: w324 -> [_ _ w326]
          frame "False", Default {
          }
          frame "True" {
          }
          frame "Mixed" {
            n191 = property class="XYGraph (strict)"(reference=w326, "Legend Visible"=FALSE ("Legend:Visible")) -> ()  [unwired: 1 in, 2 out]
          }
        }
      }
      event "XY Graph": Scale Range Change {
        n192 = event-data() -> ("CtlRef"=w329:refnum<vi>)  [unwired: 1 in]
        n193 = disable-structure shown="Disabled" {
          disable-tunnel: w329 -> [w342 _]
          disable-tunnel: [w339 w347] -> w328
          disable-tunnel: w327 -> [w336 w347]
          frame Disabled {
            n194 = while {
              tunnel: w342 -> [w346]
              tunnel: [w343] -> w341 mode=indexing
              i -> [w345]
              stop <- w344 stop-if-true
              n195 = property class="XYGraph (strict)"(reference=w346, "ActXScl"=w345) -> (error out=w344:errorcluster, "XScale.Range"=w343:T4)  [unwired: 1 in, 1 out]
            }
            n196 = Unbundle By Name(w336) -> ("state"=w335:refnum<user-event>)
            n197 = Delete From Array(array=w341) -> (array with subset deleted=w340:T4[])  [unwired: 2 in, 1 out]
            n198 = Index Array(array=w340) -> (element=w333:T4)  [unwired: 1 in]
            n199 = Generate User Event(user event=w335, event data cluster="find files" ("event data")) -> (user event out=w332:refnum<user-event>, error out=w331:errorcluster)  [unwired: 2 in]
            n200 = Bundle By Name(cluster=w336, "Settings.X Range"=w333) -> (w339:T10)
            n201 = Generate User Event(user event=w332, event data cluster="Plot All" ("event data"), error in=w331) -> ()  [unwired: 1 in, 2 out]
            n202 = Unbundle By Name(w339) -> ("Settings"=w338:T3)
            n203 = call "Rd Wr GUI Settings.vi"("Write? (F:Read)"=TRUE, "Settings"=w338) -> ()  [unwired: 8 in, 2 out]
          }
          frame Enabled {
          }
        }
      }
      event "Channel Select": Value Change {
        # "optimize by only adding new channels"
        n204 = event-data() -> ("CtlRef"=w358:refnum<vi>, "NewVal"=w356:i32[])  [unwired: 1 in]
        n205 = disable-structure shown="Enabled" {
          disable-tunnel: w354 -> [w362 w364]
          disable-tunnel: [w359 w363] -> w350
          frame Disabled {
            n206 = Unbundle By Name(w362) -> ("state"=w361:refnum<user-event>)
            n207 = Generate User Event(user event=w361, event data cluster="Plot All" ("event data")) -> (user event out=w359:refnum<user-event>)  [unwired: 2 in, 1 out]
          }
          frame Enabled {
            n208 = Unbundle By Name(w364) -> ("state"=w363:refnum<user-event>)
          }
        }
        n209 = property class="MCListbox (strict)"(reference=w358) -> ("ItemNames"=w357:string[][])  [unwired: 1 in, 2 out]
        n210 = Generate User Event(user event=w350, event data cluster="save panel position" ("event data")) -> ()  [unwired: 2 in, 2 out]
        n211 = for {
          tunnel: w357 -> [w368]
          tunnel: w356 -> [w367] mode=indexing
          tunnel: [w365] -> w355 mode=indexing
          n212 = Index Array(array=w368, index (row)=w367, index (col)=0 ("disabled index (col)")) -> (element=w365:string)
        }
        n213 = property on="XY Graph" class="XYGraph (strict)"() -> ("XScale.Range"=w348:T4)  [unwired: 2 in, 2 out]
        n214 = Bundle By Name(cluster=w354, "Settings.X Range"=w348, "Settings.Select Ch"=w355) -> (w351:T10)
        n215 = Unbundle By Name(w351) -> ("Settings"=w353:T3)
        n216 = call "Rd Wr GUI Settings.vi"("Write? (F:Read)"=TRUE, "Settings"=w353) -> ()  [unwired: 8 in, 2 out]
      }
      event "X Autoscale": Value Change {
        n217 = event-data() -> ()  [unwired: 1 in, 6 out]
        n218 = Select(t=u8 1 ("X Scale.Scale Fit"), s="X Autoscale", f=u8 0 ("X Scale.Scale Fit")) -> (s? t:f=w370:u8)
        n219 = property on="XY Graph" class="XYGraph (strict)"("ActXScl"=0 ("Active X Scale"), "XScale.ScaleFit"=w370) -> ()  [unwired: 2 in, 2 out]
      }
      event "Y Autoscale": Value Change {
        n220 = event-data() -> ()  [unwired: 1 in, 6 out]
        n221 = Select(t=u8 2 ("X Scale.Scale Fit"), s="Y Autoscale", f=u8 0 ("X Scale.Scale Fit")) -> (s? t:f=w375:u8)
        n222 = property on="XY Graph" class="XYGraph (strict)"("YScale.ScaleFit"=w375) -> ()  [unwired: 2 in, 2 out]
      }
      event "Log Y": Value Change {
        n223 = event-data() -> ()  [unwired: 1 in, 6 out]
        n224 = Select(t=u8 1 ("X Scale.Scale Fit"), s="Log Y", f=u8 0 ("X Scale.Scale Fit")) -> (s? t:f=w381:u8)
        n225 = property on="XY Graph" class="XYGraph (strict)"("ActYScl"=u8 0 ("Y Scale.Mapping Mode"), "YScale.Mapping Mode"=w381) -> ()  [unwired: 2 in, 2 out]
      }
      event "Legend Visible": Value Change {
        n226 = event-data() -> ()  [unwired: 1 in, 6 out]
        n227 = case shown="\"Mixed\"" "Legend Visible" {
          frame "False", Default {
            n228 = property on="XY Graph" class="XYGraph (strict)"("Legend Visible"=FALSE ("Legend:Visible")) -> ()  [unwired: 2 in, 2 out]
          }
          frame "Mixed" {
          }
          frame "True" {
            n229 = property on="XY Graph" class="XYGraph (strict)"("Legend Visible"=TRUE ("Legend:Visible")) -> ()  [unwired: 2 in, 2 out]
          }
        }
        n230 = Bundle By Name(cluster=w387, "Legend"="Legend Visible") -> (w388:T10)
      }
      event Panel Close {
        n231 = event-data() -> ()  [unwired: 1 in, 3 out]
        n232 = Unbundle By Name(w393) -> ("state"=w392:refnum<user-event>)
        n233 = Generate User Event(user event=w392, event data cluster="shutdown" ("event data")) -> ()  [unwired: 2 in, 2 out]
      }
    }
  }
  n234 = flat-sequence {
    tunnel: w1 -> [_]
    frame #0 {
      n235 = property class="App"() -> ("App.Kind"=w395:T15)  [unwired: 2 in, 2 out]
      n236 = Not Equal?(x=T15."Evaluation" ("y"), y=w395) -> (x != y?=w396:bool)
      n237 = Not Equal?(x=w395, y=T15."Development System") -> (x != y?=w399:bool)
      n238 = And(x=w396, y=w399) -> (x .and. y?=w397:bool)
      n239 = Quit LabVIEW(quit? (T)=w397) -> ()
    }
  }
